vi "UDPPayloadToCommand.vi"(1 "UDP Payload":string) -> (0 "Command":T1)   [LabVIEW 2021]
uses:
  CommandType.ctl
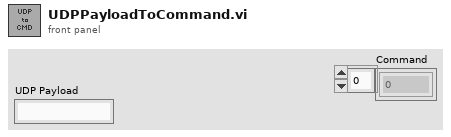
[diagram p1: front panel]
types:
  T1 = typedef "CommandType.ctl" = u8[]
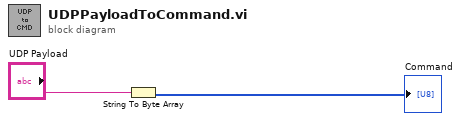
[diagram p0: block diagram]
diagram:
  n1 = String To Byte Array(string="UDP Payload") -> (unsigned byte array=→"Command":u8[])
